vi "lvEtherbone.application_example_write.vi"() -> ()   [LabVIEW 2009, in "lvEtherbone.lvlib"]
doc: "This example performs a simple write cycle to a Etherbone device."
uses:
  lvEtherbone.lvlib
panel:
  in  "data":u64=4660 format="%.0x"
  in  "address":u64=32768 format="%.0x"
  in  "ip_port":string="111.222.333.444:5555"
  out "error out":errorcluster
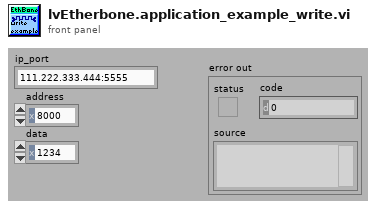
[diagram p1: front panel]
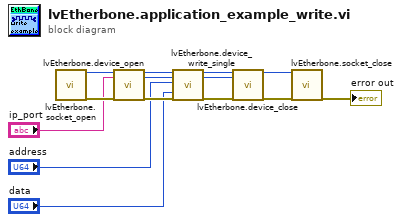
[diagram p0: block diagram]
diagram:
  n1 = call "lvEtherbone.socket_open.vi"() -> ("eb_socket_ID"=w2:i32, "error out"=w13:errorcluster)  [unwired: 17 in, 1 out]
  n2 = call "lvEtherbone.device_open.vi"("eb_socket_ID"=w2, "ip_port"="ip_port", "error in (no error)"=w13) -> ("eb_socket_ID out"=w1:i32, "eb_device_ID"=w11:i32, "error out"=w12:errorcluster)  [unwired: 13 in, 1 out]
  n3 = call "lvEtherbone.device_write_single.vi"("eb_socketID"=w1, "eb_deviceID"=w11, "address"="address", "data"="data", "error in (no error)"=w12) -> ("eb_socketID out"=w5:i32, "eb_deviceID out"=w4:i32, "error out"=w3:errorcluster)  [unwired: 11 in, 1 out]
  n4 = call "lvEtherbone.device_close.vi"("eb_socket_ID"=w5, "eb_device_ID"=w4, "error in (no error)"=w3) -> ("eb_socket_ID out"=w7:i32, "error out"=w10:errorcluster)  [unwired: 14 in, 1 out]
  n5 = call "lvEtherbone.socket_close.vi"("eb_socket_ID"=w7, "error in (no error)"=w10) -> ("error out"=→"error out":errorcluster)  [unwired: 16 in, 1 out]
